vi "Make Unique Node Name.vi"(10 "Node Name":string, 11 "CI Serializer in":refnum<class "CI Serializer.lvclass">) -> (2 "Unique Node Name":string)   [LabVIEW 2014, in "CI Serializer.lvclass"]
uses:
  CI Serializer.lvclass
  CI Serializer.lvclass/CI Serializer.ctl
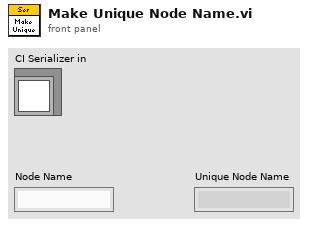
[diagram p1: front panel]
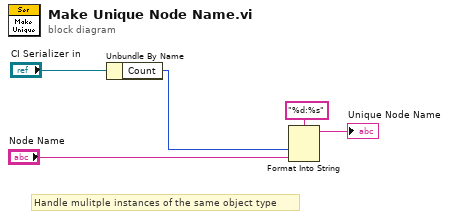
[diagram p0: block diagram]
diagram:
  # "Handle mulitple instances of the same object type"
  n1 = Unbundle By Name("CI Serializer in") -> ("Count"=w3:i32)
  n2 = Format Into String(format string="%d:%s", w3, "Node Name") -> (resulting string=→"Unique Node Name":string)  [unwired: 2 in, 1 out]
